vi "Generate Error.vi"(8 "Error In":errorcluster, 11 "Error Type":T1) -> (0 "Error Out":errorcluster)   [LabVIEW 2011, in "LVH-Adept.lvlib"]
uses:
  LVH-Adept.lvlib
  Type Defs/Error Type.ctl
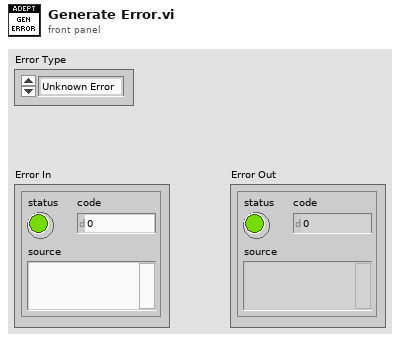
[diagram p1: front panel]
types:
  T1 = typedef "LVH-Adept.lvlib/Error Type.ctl" = enum16{"Unknown Error", "Device Enumeration", "Device Handle", "Device Info"}
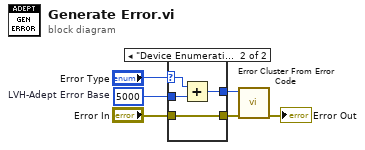
[diagram p0: block diagram]
diagram:
  w5 = 5000  # LVH-Adept Error Base
  n1 = case shown="\"Device Enumeration\"" "Error Type" {
    selector: "Error Type" -> [_ w12]
    tunnel: w5 -> [w8 w11]
    tunnel: [w8 w10] -> w4
    tunnel: "Error In" -> [w7 w9]
    tunnel: [w7 w9] -> w1
    frame "Unknown Error", Default {
    }
    frame "Device Enumeration" {
      n2 = Add(x=w12, y=w11) -> (x+y=w10:i32)
    }
  }
  n3 = call <vilib>:"Error Cluster From Error Code.vi"("error in (no error)"=w1, "error code (0)"=w4) -> ("error out"=→"Error Out":errorcluster)  [unwired: 7 in]
